vi "Start.vi"(8 "error in (no error)":errorcluster, 11 "Integrator in":refnum<class "Integrator.lvclass">) -> (0 "error out":errorcluster, 3 "Integrator out":refnum<class "Integrator.lvclass">)   [LabVIEW 2016, in "Integrator.lvclass"]
uses:
  Integrator.lvclass
  Integrator.lvclass/Integrator.ctl
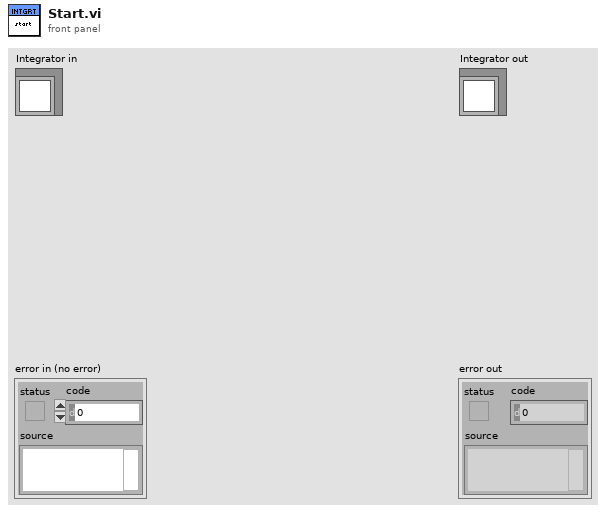
[diagram p1: front panel]
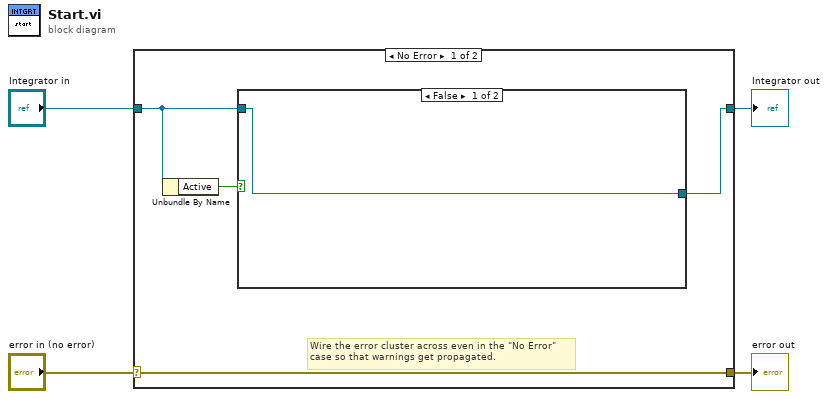
[diagram p0: block diagram]
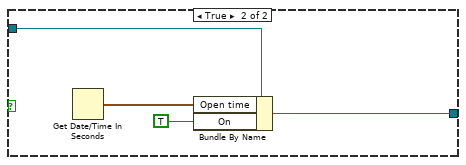
[diagram p2: hidden frame]
diagram:
  n1 = case shown="No Error" "error in (no error)" {
    selector: "error in (no error)" -> [w8 w15]
    tunnel: [w8 w15] -> w3
    tunnel: [w7 w14] -> w1
    tunnel: "Integrator in" -> [w6 w14]
    frame No Error {
      # "Wire the error cluster across even in the \"No Error\"\ncase so that warnings get propagated."
      n2 = Unbundle By Name(w6) -> ("Active"=w5:bool)
      n3 = case shown="False" w5 {
        tunnel: w6 -> [w9 w13]
        tunnel: [w9 w12] -> w7
        frame False {
        }
        frame True {
          n4 = Get Date/Time In Seconds() -> (seconds since 1Jan1904=w11:timestamp)
          n5 = Bundle By Name(cluster=w13, "Open time"=w11, "On"=TRUE) -> (w12:refnum<class "Integrator.lvclass">)
        }
      }
    }
    frame Error {
    }
  }
  "error out" <- w3
  "Integrator out" <- w1
